vi "JKISM++ TCP Server SubModule(Beside Loop Support).vi"(7 "Name(\"\" to use uuid)":string="Event JKISM Tiny") -> ()   [LabVIEW 2014]
doc: "Demonstrates how to set up a basic TCP connection, send data to the specified port once a connection has been established, and terminate the connection once the data has been sent. This VI is designed to stop if the TCP connection is terminated. The data sent in this example is an array of random numbers."
uses:
  user.lib/_NEVSTOP/JKI State Machine++/_Support/JKISMQ/_Create Data Queue.vi
  user.lib/_NEVSTOP/JKI State Machine++/_Support/JKISMQ/_Obtain JKISMQ.vi
  user.lib/_NEVSTOP/JKI State Machine++/_Support/FGV-BroadcastRegistry/Cache-Broadcast Registry Search Result.vi
  user.lib/_NEVSTOP/JKI State Machine++/AdvanceAPI/JKISM++ Register Status Change.vi
  user.lib/_NEVSTOP/JKI State Machine++/AdvanceAPI/JKISM++ Unregister Status Change.vi
  user.lib/_NEVSTOP/JKI State Machine++/_Support/JKISMQ/_Create Resp Queue.vi
  user.lib/_NEVSTOP/JKI State Machine++/_Support/JKISMQ/_Unlock JKISMQ.vi
  user.lib/_NEVSTOP/JKI State Machine++/_Support/JKISMQ/_Lock State JKISMQ.vi
  user.lib/_NEVSTOP/JKI State Machine++/_Support/JKISMQ/_Release JKISMQ.vi
  user.lib/_NEVSTOP/JKI State Machine++/AdvanceAPI/JKISM++ Make String Arguments Safe.vi
  user.lib/_NEVSTOP/JKI State Machine++/_Support/JKISMQ/_Input Name to JKISM Mode.vi
  user.lib/_NEVSTOP/JKI State Machine++/Utility/uuid.vi
  user.lib/_NEVSTOP/JKI State Machine++/_Support/KeyWords.vi
  user.lib/_NEVSTOP/JKI State Machine++/_Support/JKISMQ/_JKISMQFGV.vi
  user.lib/_NEVSTOP/JKI State Machine++/_Support/GlobalEvent/FGV-GlobalEventRef.vi
  user.lib/_NEVSTOP/JKI State Machine++/_Support/JKISMQ/_Dequeue JKISMQ.vi
  user.lib/_NEVSTOP/JKI State Machine++/_Support/JKISMQ/_Enqueue JKISMQ.vi
  user.lib/_NEVSTOP/JKI State Machine++/_Support/GlobalEvent/FGV-StatusChangeEventRef.vi
  user.lib/_NEVSTOP/JKI State Machine++/_Support/FGV-BroadcastRegistry/global-Broadcast Cache Change Flag.vi
  user.lib/_NEVSTOP/JKI State Machine++/_Support/FGV-BroadcastRegistry/FGV-BroadcastRegistry.vi
  user.lib/_NEVSTOP/JKI State Machine++/JKI State Machine++.lvlib
panel:
  in  "Send String":string
  out "Connected":bool
  out "TCP Received":string
  out "TCP":refnum<k5>
  out "State History":string
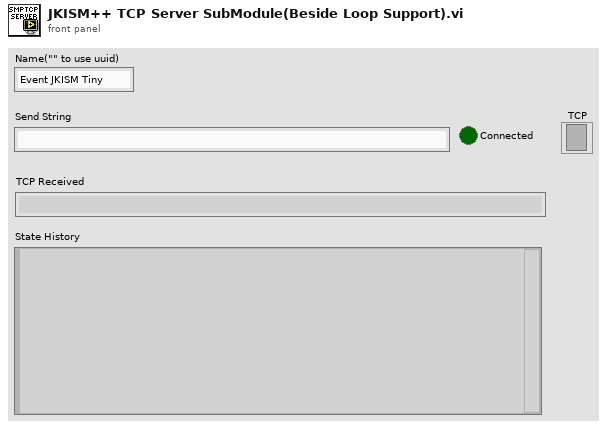
[diagram p1: front panel]
types:
  T1 = enum32{"Invalid", "Standard", "Closed", "Hidden", "Minimized", "Maximized"}
  T2 = enum32{"invalid app kind", "Development System", "Run Time System", "Student Edition", "Embedded LabVIEW", "Evaluation", "Custom"}
  T3 = cluster{"Core":cluster{"Current VI Reference":refnum<vi>, "Close Panel on Exit?":bool}, "Your Boolean data":bool, "Your string data":string}
  T4 = cluster{"Current VI Reference":refnum<vi>, "Close Panel on Exit?":bool}
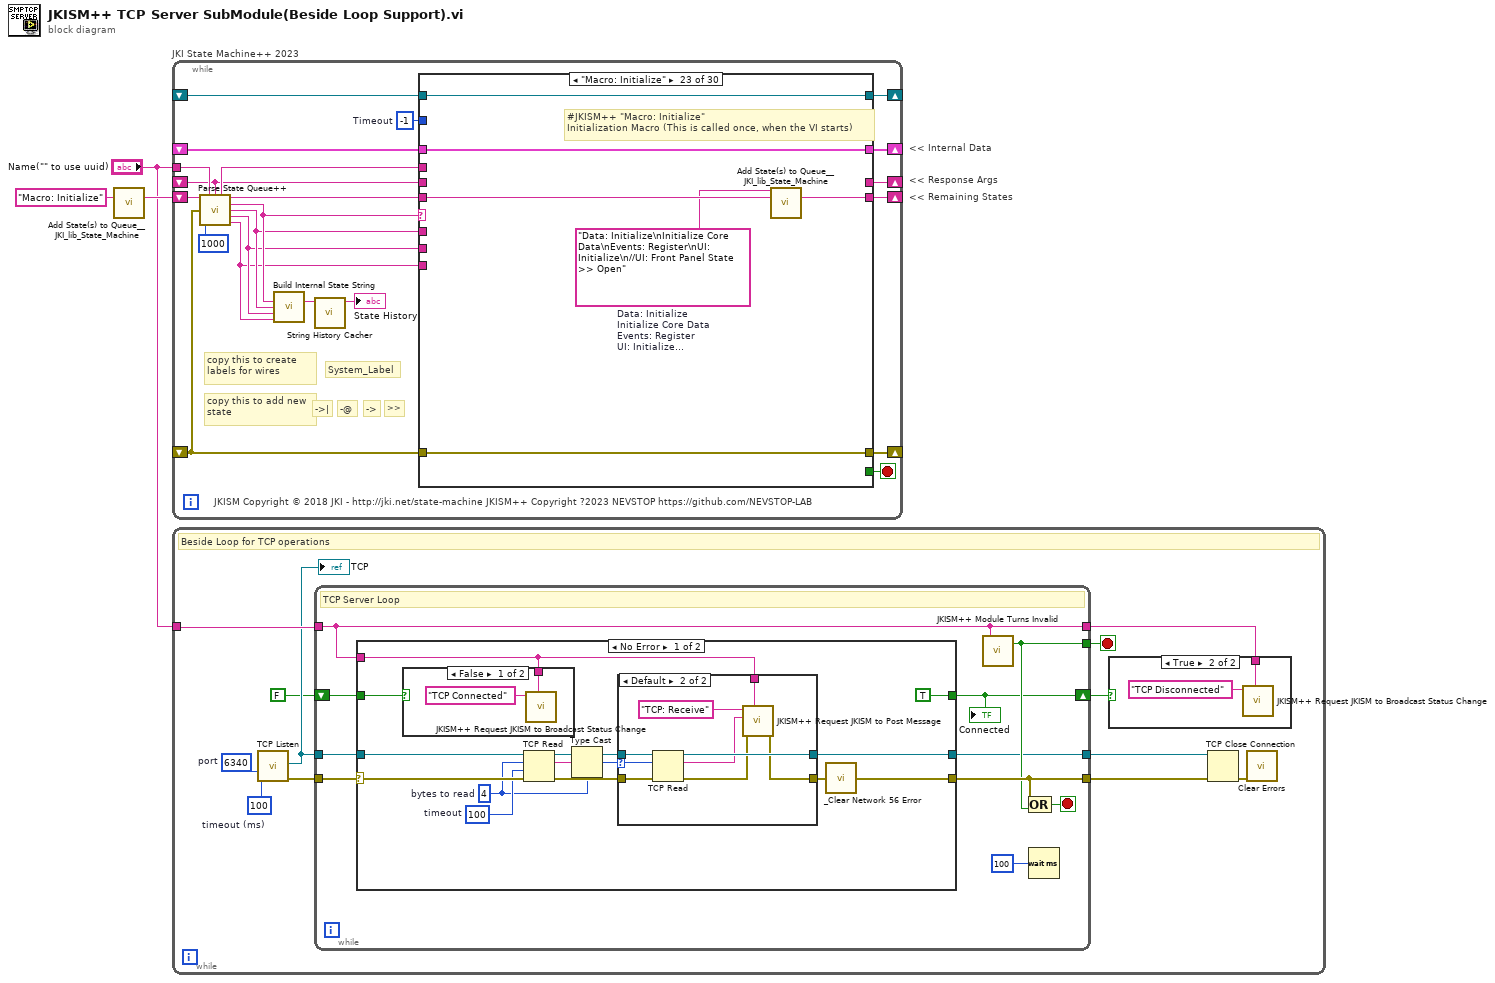
[diagram p0: block diagram]
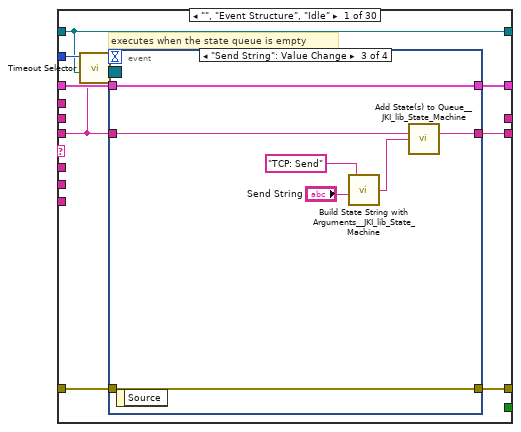
[diagram p2: hidden frame]
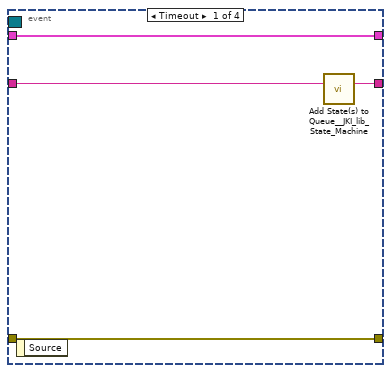
[diagram p3: hidden frame]
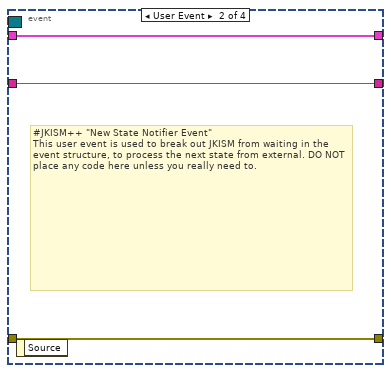
[diagram p4: hidden frame]
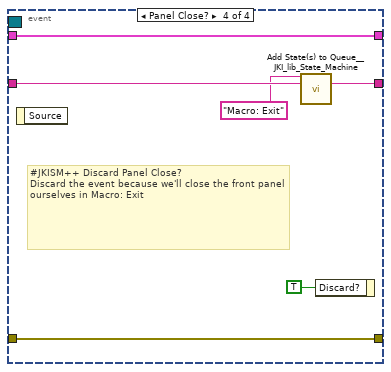
[diagram p5: hidden frame]
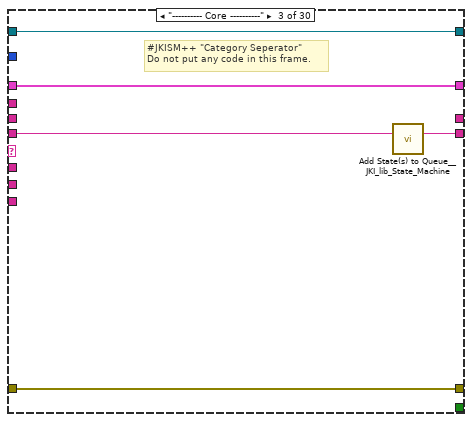
[diagram p7: hidden frame]
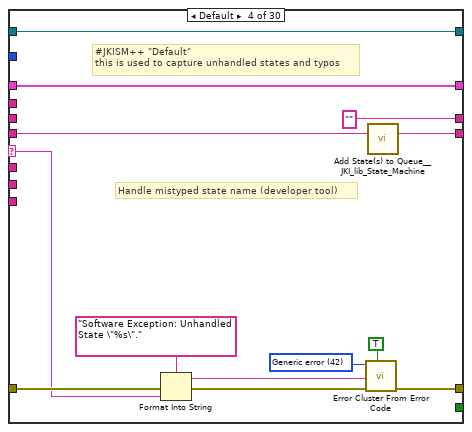
[diagram p8: hidden frame]
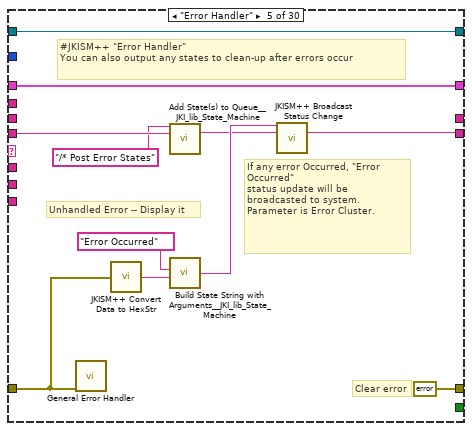
[diagram p9: hidden frame]
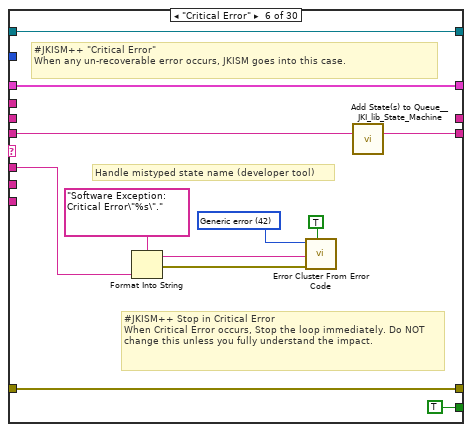
[diagram p10: hidden frame]
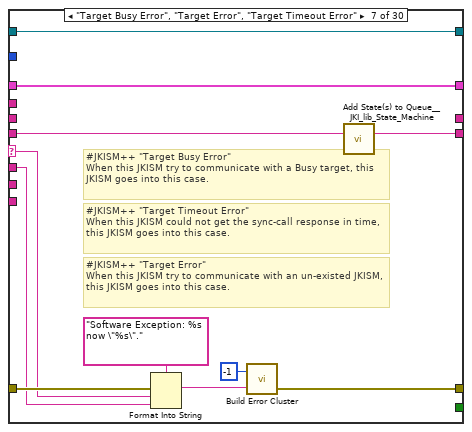
[diagram p11: hidden frame]
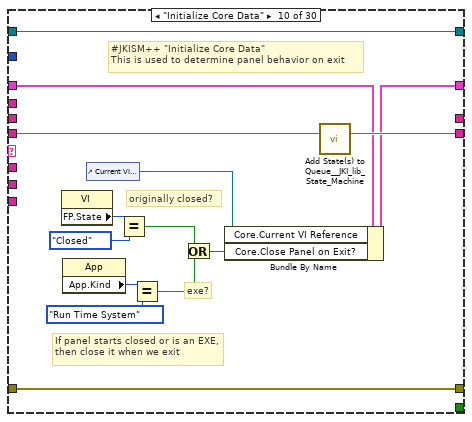
[diagram p14: hidden frame]
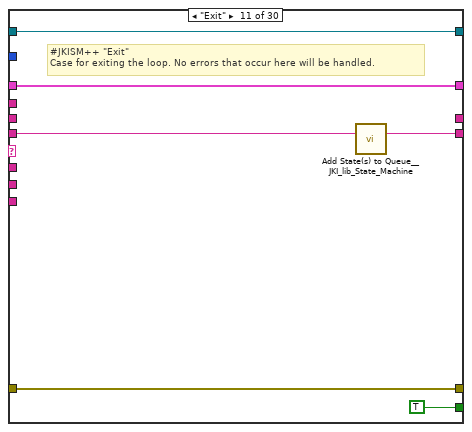
[diagram p15: hidden frame]
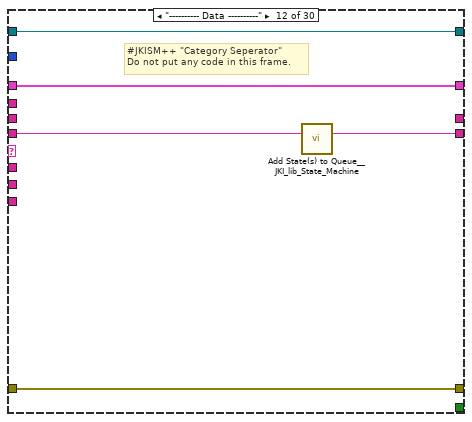
[diagram p16: hidden frame]
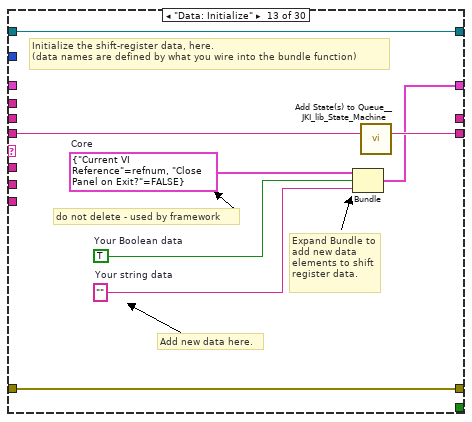
[diagram p17: hidden frame]
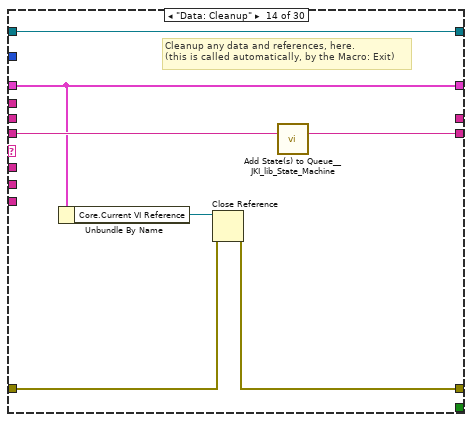
[diagram p18: hidden frame]
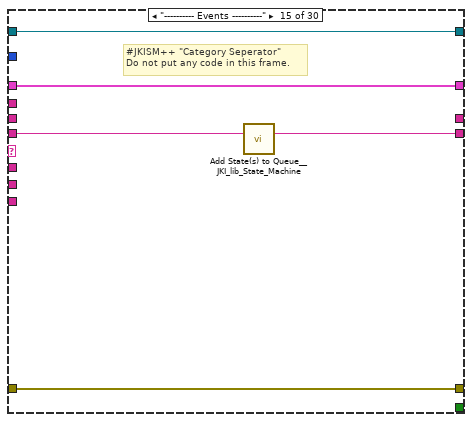
[diagram p19: hidden frame]
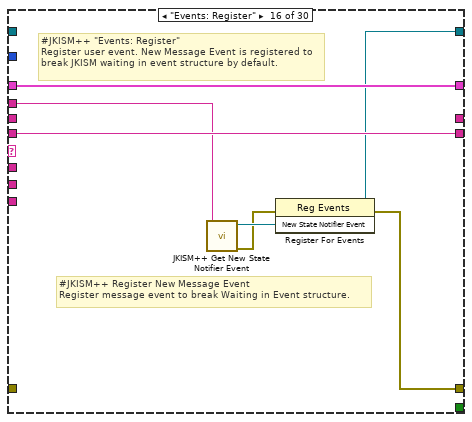
[diagram p20: hidden frame]
diagram:
  # "<< Internal Data"
  # "<< Response Args"
  # "<< Remaining States"
  n1 = call <vilib>:"Add State(s) to Queue__JKI_lib_State_Machine.vi"("State(s) in (\"\")"="Macro: Initialize") -> ("States Out"=w2:string)  [unwired: 14 in]
  n2 = while "JKI State Machine++ 2023" {
    shift-right: [w20] -> _
    shift-left: _ -> [w19]
    shift-right: [w23] -> _
    shift-left: _ -> [w17]
    shift-right: [w22] -> _
    shift-left: w2 -> [w24]
    tunnel: "Name(\"\" to use uuid)" -> [w12]
    shift-right: [w15] -> _
    shift-left: _ -> [w4]
    shift-right: [w14] -> _
    shift-left: _ -> [w13]
    stop <- w21 stop-if-true
    w18 = -1  # Timeout
    # "->|"
    # "JKISM Copyright © 2018 JKI - http://jki.net/state-machine JKISM++ Copyright ?2023 NEVSTOP https://github.com/NEVSTOP-LAB"
    # "copy this to add new state"
    # ">>"
    # "->"
    # "-@"
    # "copy this to create labels for wires"
    # "System_Label"
    n3 = call "Parse State Queue++.vi"("State Queue"=w24, "Name(\"\" to use uuid)"=w12, "Response Arguments"=w4, "Error In (no error)"=w17, "Response Timeout(5000ms)"=1000 ("Response Timeout(1000ms)")) -> ("Name Used"=w5:string, "Remaining States"=w25:string, "Current State"=w9:string, "Arguments"=w8:string, "Argument - State"=w7:string, "From Who"=w6:string)  [unwired: 5 in]
    n4 = call "Build Internal State String.vi"("State"=w9, "Arguments (\"\")"=w8, "Arg-State (\"\")"=w7, "Source (\"\")"=w6) -> ("State with Arguments"=w10:string)  [unwired: 11 in]
    n5 = call "String History Cacher.vi"("String"=w10) -> ("String Cache"=→"State History":string)  [unwired: 10 in]
    n6 = case shown="\"Macro: Initialize\"" w9 {
      selector: w9 -> [_ _ _ w66 _ _ w103 _ _ _ _ _ _ _ _ _ _ _ _ _ _ _ _ _ _ _ _ _ _ _]
      tunnel: w25 -> [w26 w57 w63 w70 w87 w97 w105 w113 w117 w132 w138 w143 w151 w158 w163 w170 w174 w180 w185 w192 w208 w278 w284 w295 w298 w309 w316 w322 w328 w334]
      tunnel: w8 -> [_ _ _ _ _ w90 w104 _ _ _ _ _ _ _ _ _ _ _ _ w187 w202 _ _ _ _ w300 w311 _ _ _]
      tunnel: w19 -> [w33 w56 w60 w68 w85 w98 w107 w112 w116 w125 w136 w140 _ w153 w160 w169 w173 w177 w183 w190 w204 w275 w281 w292 w297 w308 w315 w319 w325 w331]
      tunnel: [w32 w58 w61 w72 errorcluster {"status"=FALSE, "code"=0, "source"=""} ("error out") w99 w101 w114 w118 w129 w135 w141 w148 w154 w161 w164 w172 w178 w182 w188 w205 w276 w282 w293 w299 w301 w317 w320 w326 w332] -> w23
      tunnel: w17 -> [w31 w58 w61 w71 w77 w99 w109 w114 w118 w129 w135 w141 w148 w155 w161 _ w175 w178 w182 w189 w206 w276 w282 w293 w299 _ w317 w320 w326 w332]
      tunnel: [w34 w57 w62 w69 w78 w96 w108 w113 w117 w131 w137 w142 w150 w157 w162 w170 w174 w179 w184 w191 w207 w277 w283 w294 w298 w309 w313 w321 w327 w333] -> w22
      tunnel: [_ _ _ _ _ TRUE _ _ _ _ TRUE _ _ _ _ _ _ _ _ _ _ _ _ _ _ _ _ _ _ _] -> w21
      tunnel: [w30 w56 w60 w68 w85 w98 w107 w112 w116 w130 w136 w140 w149 w153 w160 w169 w173 w177 w183 w190 w204 w275 w281 w292 w297 w308 w315 w319 w325 w331] -> w20
      tunnel: w18 -> [w29 _ _ _ _ _ _ _ _ _ _ _ _ _ _ _ _ _ _ _ _ _ _ _ _ _ _ _ _ _]
      tunnel: w6 -> [_ _ _ _ _ _ _ _ _ _ _ _ _ _ _ _ _ _ _ _ _ _ _ _ _ _ _ _ _ _]
      tunnel: w7 -> [_ _ _ _ _ _ _ _ _ _ _ _ _ _ _ _ _ _ _ _ _ _ _ _ _ _ _ _ _ _]
      tunnel: [_ _ _ "" _ _ _ _ _ _ _ _ _ _ _ _ _ _ _ _ _ _ _ _ _ _ _ _ "DoA Finished" "DoB Finished"] -> w15
      tunnel: [w28 w55 w59 w64 w83 w88 w106 w111 w115 w119 w133 w139 w144 w152 w159 w168 w171 w176 w181 w186 w201 w274 w279 w285 w296 w307 w314 w318 w324 w330] -> w14
      tunnel: w13 -> [w28 w55 w59 w64 w83 w88 w106 w111 w115 w119 w133 w139 w144 w152 w159 _ w171 w176 w181 w186 w201 w274 w279 w285 w296 w307 w314 w318 w324 w330]
      tunnel: w5 -> [_ _ _ _ _ _ _ _ _ _ _ _ _ _ _ w167 _ _ _ _ _ _ _ _ _ _ _ _ _ _]
      tunnel: w4 -> [_ _ _ _ _ _ _ _ _ _ _ _ _ _ _ _ _ _ _ _ _ _ _ _ _ _ _ _ _ _]
      frame "", "Event Structure", "Idle" {
        # "executes when the state queue is empty"
        n7 = call "Timeout Selector.vi"("Remaining States"=w26, "Timeout Expected"=w29) -> ("Timeout"=w27:i32)  [unwired: 5 in]
        n8 = event shown="[2] \"Send String\": Value Change" {
          selector: w28 -> [_ _ _ _]
          dyn-events: _ -> [_ _ _ _]
          timeout: w27 -> [_ _ _ _]
          tunnel: w26 -> [w38 w40 w46 w54]
          tunnel: [w37 w40 w45 w53] -> w34
          tunnel: w33 -> [w35 w41 w47 w51]
          tunnel: [w36 w39 w48 w52] -> w32
          tunnel: w31 -> [w36 w39 w48 w52]
          tunnel: [w35 w41 w47 w51] -> w30
          event Timeout {
            n9 = event-data() -> ()  [unwired: 1 in, 1 out]
            n10 = call <vilib>:"Add State(s) to Queue__JKI_lib_State_Machine.vi"("State(s) in (\"\")"=w38) -> ("States Out"=w37:string)  [unwired: 14 in]
          }
          event User Event {
            # "#JKISM++ \"New State Notifier Event\"\nThis user event is used to break out JKISM from waiting in the event structure, to process the next state from external. DO NOT place any code here unless you really need to."
            n11 = event-data() -> ()  [unwired: 1 in, 1 out]
          }
          event "Send String": Value Change {
            n12 = event-data() -> ()  [unwired: 1 in, 1 out]
            n13 = call <vilib>:"Build State String with Arguments__JKI_lib_State_Machine.vi"("Arguments (\"\")"="Send String", "State"="TCP: Send") -> ("State with Arguments"=w43:string)  [unwired: 4 in]
            n14 = call <vilib>:"Add State(s) to Queue__JKI_lib_State_Machine.vi"("State(s) in (\"\")"=w46, "State(s) at Back (\"\")"=w43) -> ("States Out"=w45:string)  [unwired: 13 in]
          }
          event Panel Close? {
            # "#JKISM++ Discard Panel Close?\nDiscard the event because we'll close the front panel ourselves in Macro: Exit"
            n15 = event-data() -> ()  [unwired: 1 in, 1 out]
            n16 = call <vilib>:"Add State(s) to Queue__JKI_lib_State_Machine.vi"("State(s) in Front (\"\")"="Macro: Exit", "State(s) in (\"\")"=w54) -> ("States Out"=w53:string)  [unwired: 13 in]
            n17 = event-data("Discard?"=TRUE) -> ()  [unwired: 1 in, 1 out]
          }
        }
      }
      frame "JKISM++ Documentation" {
        # "#JKISM++ \"Documentation\"\nCase for holding JKISM++ Documenation"
      }
      frame "---------- Core ----------" {
        # "#JKISM++ \"Category Seperator\"\nDo not put any code in this frame."
        n18 = call <vilib>:"Add State(s) to Queue__JKI_lib_State_Machine.vi"("State(s) in (\"\")"=w63) -> ("States Out"=w62:string)  [unwired: 14 in]
      }
      frame Default {
        w75 = 42 items=["No error", "Argument error", "Memory is full", "Out of zone", "End of file", "File already open", "Generic file I/O error", "File not found", "File permission error", "Disk is full", "Duplicate path", "Too many files open", "System feature not enabled", "Resource file not found", "Cannot add resource", "Resource not found", "Image not found", "Image memory error", "Pen does not exist", "Config type invalid", "Config token not found", "Config parse error", "Config memory error", "Bad external code format", "Bad external code offset", "External code not present", "Null window", "Destroy window error", "Null menu", "Print aborted", "Bad print record", "Print driver error", "Windows error during printing", "Memory error during printing", "Print dialog error", "Generic print error", "Invalid device refnum", "Device not found", "Device parameter error", "Device unit error", "Cannot open device", "Device call aborted", "Generic error", "Cancelled by user", "Object ID too low", "Object ID too high", "Object not in heap", "Unknown heap", "Unknown object (invalid DefProc)", "Unknown object (DefProc not in table)", "Message out of range", "Invalid (null) method", "Unknown message", "Manager call not supported", "Bad address", "Network operation in progress", "Network operation timed out", "Connection is busy", "Network attribute not supported", "Network error", "Address in use", "System out of memory", "Connection aborted", "Connection refused", "Not connected", "Already connected", "Connection closed", "Initialization error (interapplication manager)", "Bad occurrence", "Wait on unbound occurrence handler", "Occurrence queue overflow", "Datalog type conflict", "Unused", "Unrecognized type (interapplication manager)", "Memory corrupt", "Failed to make temporary DLL", "Old CIN version", "Drag socket not found", "Failed to load drop-object", "Failed to register OLE object", "Failed to release OLE object", "Format specifier type mismatch", "Unknown format specifier", "Too few format specifiers", "Too many format specifiers", "Scan failed", "Newer CIN version", "Error converting to variant", "Runtime menu error", "Password tampered", "Variant attribute not found", "Incompatible variant data type", "Event data is not available", "Event Store is not present", "Occurrence is not found", "Event Queue is not created", "Event info is not available", "Refnum passed is NULL", "Error retrieving Class GUID", "Error retrieving CoClass GUID", "Error retrieving TypeLib GUID.", "Bad built application magic bytes.", "Specific driver is different from the specific driver associated with the Logical Name.", "There is no session opened to the class driver.", "Max Error", "MAX - Error with config objects", "MAX - Error loading configuration", "MAX - Group not supported"]
        # "#JKISM++ \"Default\"\nthis is used to capture unhandled states and typos"
        # "Handle mistyped state name (developer tool)"
        n19 = Format Into String(format string="Software Exception: Unhandled State \"%s\"." ("message"), error in=w71, w66) -> (resulting string=w74:string, error out=w73:errorcluster)  [unwired: 1 in]
        n20 = call <vilib>:"Error Cluster From Error Code.vi"("show call chain? (False)"=TRUE, "error in (no error)"=w73, "error message (\"\")"=w74, "error code (0)"=w75) -> ("error out"=w72:errorcluster)  [unwired: 5 in]
        n21 = call <vilib>:"Add State(s) to Queue__JKI_lib_State_Machine.vi"("State(s) in (\"\")"=w70) -> ("States Out"=w69:string)  [unwired: 14 in]
      }
      frame "Error Handler" {
        # "#JKISM++ \"Error Handler\"\nYou can also output any states to clean-up after errors occur"
        # "If any error Occurred, \"Error Occurred\" \nstatus update will be broadcasted to system.\nParameter is Error Cluster."
        # "Unhandled Error -- Display it"
        # "Clear error"
        n22 = call <vilib>:"General Error Handler.vi"("error in (no error)"=w77) -> ()  [unwired: 10 in, 5 out]
        n23 = call "JKISM++ Convert Data to HexStr.vi"("Variant"=w77) -> ("HEX String (0-9,A-F)"=w81:string)  [unwired: 8 in]
        n24 = call <vilib>:"Add State(s) to Queue__JKI_lib_State_Machine.vi"("State(s) in Front (\"\")"="/* Post Error States", "State(s) in (\"\")"=w87) -> ("States Out"=w79:string)  [unwired: 13 in]
        n25 = call <vilib>:"Build State String with Arguments__JKI_lib_State_Machine.vi"("Arguments (\"\")"=w81, "State"="Error Occurred" ("Status with Arguments")) -> ("State with Arguments"=w80:string)  [unwired: 4 in]
        n26 = call "JKISM++ Broadcast Status Change.vi"("Status with Arguments"=w80, "State Queue"=w79) -> ("Remaining States"=w78:string)  [unwired: 13 in]
      }
      frame "Critical Error" {
        w94 = 42 items=["No error", "Argument error", "Memory is full", "Out of zone", "End of file", "File already open", "Generic file I/O error", "File not found", "File permission error", "Disk is full", "Duplicate path", "Too many files open", "System feature not enabled", "Resource file not found", "Cannot add resource", "Resource not found", "Image not found", "Image memory error", "Pen does not exist", "Config type invalid", "Config token not found", "Config parse error", "Config memory error", "Bad external code format", "Bad external code offset", "External code not present", "Null window", "Destroy window error", "Null menu", "Print aborted", "Bad print record", "Print driver error", "Windows error during printing", "Memory error during printing", "Print dialog error", "Generic print error", "Invalid device refnum", "Device not found", "Device parameter error", "Device unit error", "Cannot open device", "Device call aborted", "Generic error", "Cancelled by user", "Object ID too low", "Object ID too high", "Object not in heap", "Unknown heap", "Unknown object (invalid DefProc)", "Unknown object (DefProc not in table)", "Message out of range", "Invalid (null) method", "Unknown message", "Manager call not supported", "Bad address", "Network operation in progress", "Network operation timed out", "Connection is busy", "Network attribute not supported", "Network error", "Address in use", "System out of memory", "Connection aborted", "Connection refused", "Not connected", "Already connected", "Connection closed", "Initialization error (interapplication manager)", "Bad occurrence", "Wait on unbound occurrence handler", "Occurrence queue overflow", "Datalog type conflict", "Unused", "Unrecognized type (interapplication manager)", "Memory corrupt", "Failed to make temporary DLL", "Old CIN version", "Drag socket not found", "Failed to load drop-object", "Failed to register OLE object", "Failed to release OLE object", "Format specifier type mismatch", "Unknown format specifier", "Too few format specifiers", "Too many format specifiers", "Scan failed", "Newer CIN version", "Error converting to variant", "Runtime menu error", "Password tampered", "Variant attribute not found", "Incompatible variant data type", "Event data is not available", "Event Store is not present", "Occurrence is not found", "Event Queue is not created", "Event info is not available", "Refnum passed is NULL", "Error retrieving Class GUID", "Error retrieving CoClass GUID", "Error retrieving TypeLib GUID.", "Bad built application magic bytes.", "Specific driver is different from the specific driver associated with the Logical Name.", "There is no session opened to the class driver.", "Max Error", "MAX - Error with config objects", "MAX - Error loading configuration", "MAX - Group not supported"]
        # "#JKISM++ Stop in Critical Error\nWhen Critical Error occurs, Stop the loop immediately. Do NOT change this unless you fully understand the impact."
        # "#JKISM++ \"Critical Error\"\nWhen any un-recoverable error occurs, JKISM goes into this case."
        # "Handle mistyped state name (developer tool)"
        n27 = Format Into String(format string="Software Exception: Critical Error\"%s\"." ("message"), w90) -> (resulting string=w93:string, error out=w92:errorcluster)  [unwired: 2 in]
        n28 = call <vilib>:"Error Cluster From Error Code.vi"("show call chain? (False)"=TRUE, "error in (no error)"=w92, "error message (\"\")"=w93, "error code (0)"=w94) -> ()  [unwired: 5 in, 1 out]
        n29 = call <vilib>:"Add State(s) to Queue__JKI_lib_State_Machine.vi"("State(s) in (\"\")"=w97) -> ("States Out"=w96:string)  [unwired: 14 in]
      }
      frame "Target Busy Error", "Target Error", "Target Timeout Error" {
        # "#JKISM++ \"Target Error\"\nWhen this JKISM try to communicate with an un-existed JKISM, this JKISM goes into this case."
        # "#JKISM++ \"Target Timeout Error\"\nWhen this JKISM could not get the sync-call response in time, this JKISM goes into this case."
        # "#JKISM++ \"Target Busy Error\"\nWhen this JKISM try to communicate with a Busy target, this JKISM goes into this case."
        n30 = Format Into String(format string="Software Exception: %s now \"%s\"." ("message"), error in=w109, w103, w104) -> (resulting string=w102:string)  [unwired: 1 in, 1 out]
        n31 = call "Build Error Cluster.vi"("String to Prepend to source (\"\")"=w102, "code"=-1) -> ("error out"=w101:errorcluster)
        n32 = call <vilib>:"Add State(s) to Queue__JKI_lib_State_Machine.vi"("State(s) in (\"\")"=w105) -> ("States Out"=w108:string)  [unwired: 14 in]
      }
      frame "Async Response", "Response" {
        # "#JKISM++ Response Comments\nAfter Message is executed, JKISM+ goes to this state for receive the response.\n    For Async Message(->), \"Async Response\" is used. This JKISM will goes to \"Async Message Posted\" immediately and receive the \"Async Response\" after the callee finishes the message.\n    For Sync Message(@),  This JKISM will wait until the message is done and immediately goes to \"Response\""
        # "#JKISM++ \"Async Response\"\nHandle Async-call Response (\"Async Response\" for ->)"
        # "#JKISM++ \"Response\"\nHandle Sync-call Response (\"Response\" for -@)"
      }
      frame "Async Message Posted" {
        # "#JKISM++ \"Async Message Posted\"\nAfter Async Message is posted (-> or ->| ), JKISM+ goes to this state for post-action.\nYou can use Argument - State to tell which Async Message is called."
      }
      frame "Initialize Core Data" {
        # "#JKISM++ \"Initialize Core Data\"\nThis is used to determine panel behavior on exit"
        # "originally closed?"
        # "exe?"
        # "If panel starts closed or is an EXE, then close it when we exit"
        n33 = property class="VI"() -> ("FP.State"=w122:T1)  [unwired: 2 in, 2 out]
        n34 = property class="App"() -> ("App.Kind"=w128:T2)  [unwired: 2 in, 2 out]
        n35 = control-ref of="Current VI Reference"() -> (w123:refnum<vi>)
        n36 = Equal?(x=w122, y=T1."Closed" ("Front Panel Window:State")) -> (x = y?=w120:bool)
        n37 = Equal?(x=w128, y=T2."Run Time System" ("Application:Kind")) -> (x = y?=w126:bool)
        n38 = Or(x=w120, y=w126) -> (x .or. y?=w124:bool)
        n39 = Bundle By Name(cluster=w125, "Core.Current VI Reference"=w123, "Core.Close Panel on Exit?"=w124) -> (w130:T3)
        n40 = call <vilib>:"Add State(s) to Queue__JKI_lib_State_Machine.vi"("State(s) in (\"\")"=w132) -> ("States Out"=w131:string)  [unwired: 14 in]
      }
      frame "Exit" {
        # "#JKISM++ \"Exit\"\nCase for exiting the loop. No errors that occur here will be handled."
        n41 = call <vilib>:"Add State(s) to Queue__JKI_lib_State_Machine.vi"("State(s) in (\"\")"=w138) -> ("States Out"=w137:string)  [unwired: 14 in]
      }
      frame "---------- Data ----------" {
        # "#JKISM++ \"Category Seperator\"\nDo not put any code in this frame."
        n42 = call <vilib>:"Add State(s) to Queue__JKI_lib_State_Machine.vi"("State(s) in (\"\")"=w143) -> ("States Out"=w142:string)  [unwired: 14 in]
      }
      frame "Data: Initialize" {
        w145 = T4 {"Current VI Reference"=refnum, "Close Panel on Exit?"=FALSE}  # Core
        w147 = TRUE  # Your Boolean data
        w146 = ""  # Your string data
        # "do not delete - used by framework"
        # "Expand Bundle to add new data elements to shift register data."
        # "Add new data here."
        # "Initialize the shift-register data, here.\n(data names are defined by what you wire into the bundle function)"
        n43 = Bundle("Core"=w145, "Your Boolean data"=w147, "Your string data"=w146) -> (w149:T3)  [unwired: 1 in]
        n44 = call <vilib>:"Add State(s) to Queue__JKI_lib_State_Machine.vi"("State(s) in (\"\")"=w151) -> ("States Out"=w150:string)  [unwired: 14 in]
      }
      frame "Data: Cleanup" {
        # "Cleanup any data and references, here.\n(this is called automatically, by the Macro: Exit)"
        n45 = Unbundle By Name(w153) -> ("Core.Current VI Reference"=w156:refnum<vi>)
        n46 = Close Reference(reference=w156, error in (no error)=w155) -> (error out=w154:errorcluster)
        n47 = call <vilib>:"Add State(s) to Queue__JKI_lib_State_Machine.vi"("State(s) in (\"\")"=w158) -> ("States Out"=w157:string)  [unwired: 14 in]
      }
      frame "---------- Events ----------" {
        # "#JKISM++ \"Category Seperator\"\nDo not put any code in this frame."
        n48 = call <vilib>:"Add State(s) to Queue__JKI_lib_State_Machine.vi"("State(s) in (\"\")"=w163) -> ("States Out"=w162:string)  [unwired: 14 in]
      }
      frame "Events: Register" {
        # "#JKISM++ \"Events: Register\"\nRegister user event. New Message Event is registered to break JKISM waiting in event structure by default."
        # "#JKISM++ Register New Message Event\nRegister message event to break Waiting in Event structure."
        n49 = call "JKISM++ Get New State Notifier Event.vi"("Name(\"\" to use uuid) in"=w167) -> ("Error out"=w165:errorcluster, "New State Notifier Event"=w166:refnum<user-event>)  [unwired: 9 in]
        n50 = register-events(error in=w165, w166) -> (reference out=w168:refnum<event-registration>, error out=w164:errorcluster)  [unwired: 1 in]
      }
      frame "Events: Unregister" {
        # "#JKISM++ \"Events: Unregister\"\nUnregister user event."
        n51 = Unregister For Events(event registration refnum=w171, error in=w175) -> (error out=w172:errorcluster)
      }
      frame "---------- UI ----------" {
        # "#JKISM++ \"Category Seperator\"\nDo not put any code in this frame."
        n52 = call <vilib>:"Add State(s) to Queue__JKI_lib_State_Machine.vi"("State(s) in (\"\")"=w180) -> ("States Out"=w179:string)  [unwired: 14 in]
      }
      frame "UI: Initialize" {
        # "#JKISM++ \"UI: Initialize\"\nInitialize the User Interface, here.\n(this is called automatically, by the Macro: Init)"
        n53 = call <vilib>:"Add State(s) to Queue__JKI_lib_State_Machine.vi"("State(s) in (\"\")"=w185) -> ("States Out"=w184:string)  [unwired: 14 in]
      }
      frame "UI: Cursor Set" {
        # "#JKISM++ \"UI: Cursor Set\"\nSet and Unset Cursor Busy.\n(Usage: \"UI: Cursor Set >> Busy|Idle\")"
        # "Argument"
        n54 = disable-structure shown="TARGET_TYPE!=Windows" {
          disable-tunnel: w189 -> [w195 w200]
          disable-tunnel: [w194 w200] -> w188
          disable-tunnel: w187 -> [w193 _]
          frame condition #0 (active) {
            n55 = case shown="\"Idle\", Default" w193 {
              tunnel: w195 -> [w197 w199]
              tunnel: [w196 w198] -> w194
              frame "Idle", Default {
                n56 = call <vilib>:"Unset Busy.vi"("error in (no error)"=w197) -> ("error out"=w196:errorcluster)  [unwired: 10 in]
              }
              frame "Busy" {
                n57 = call <vilib>:"Set Busy.vi"("error in (no error)"=w199) -> ("error out"=w198:errorcluster)  [unwired: 9 in, 1 out]
              }
            }
          }
          frame condition #1 {
          }
        }
        n58 = call <vilib>:"Add State(s) to Queue__JKI_lib_State_Machine.vi"("State(s) in (\"\")"=w192) -> ("States Out"=w191:string)  [unwired: 14 in]
      }
      frame "UI: Front Panel State" {
        # "#JKISM++ \"UI: Front Panel State\"\nSet Front Panel Open or Closed\n(Usage: \"UI: Front Panel State >> Open|Close\")"
        # "Argument"
        n59 = Unbundle By Name(w204) -> ("Core.Current VI Reference"=w203:refnum<vi>)
        n60 = call <vilib>:"Add State(s) to Queue__JKI_lib_State_Machine.vi"("State(s) in (\"\")"=w208) -> ("States Out"=w207:string)  [unwired: 14 in]
        n61 = case shown="\"Close\", \"Closed\"" w202 {
          tunnel: w206 -> [w214 w229 w240 w253 w266]
          tunnel: [w216 w230 w242 w255 w268] -> w205
          tunnel: w203 -> [w215 w227 w241 w254 w267]
          frame "Open", "Standard", Default {
            w209 = T1."Standard" ("State")
            n62 = property class="VI"(reference=w215, error in=w214) -> (reference out=w212:refnum<vi>, error out=w213:errorcluster, "FP.State"=w211:T1)
            n63 = Not Equal?(x=w211, y=w209) -> (x != y?=w210:bool)
            n64 = case shown="True" w210 {
              tunnel: [w220 w222] -> w216
              tunnel: w213 -> [w219 w222]
              tunnel: w212 -> [w218 _]
              tunnel: w209 -> [w217 _]
              frame True {
                n65 = invoke class="VI" method="FP.Open"(reference=w218, error in=w219, "Activate"=TRUE, "State"=w217) -> (error out=w220:errorcluster)  [unwired: 1 in, 4 out]
              }
              frame False {
              }
            }
          }
          frame "Close", "Closed" {
            n66 = property class="VI"(reference=w227, error in=w229) -> (reference out=w226:refnum<vi>, error out=w228:errorcluster, "FP.State"=w224:T1)
            n67 = Not Equal?(x=w224, y=T1."Closed" ("Front Panel Window:State")) -> (x != y?=w223:bool)
            n68 = case shown="False" w223 {
              tunnel: [w231 w234] -> w230
              tunnel: w228 -> [w231 w233]
              tunnel: w226 -> [_ w232]
              frame False {
              }
              frame True {
                n69 = invoke class="VI" method="FP.Close"(reference=w232, error in=w233) -> (error out=w234:errorcluster)  [unwired: 1 in, 2 out]
              }
            }
          }
          frame "Hidden", "Hide" {
            w235 = T1."Hidden" ("State")
            n70 = property class="VI"(reference=w241, error in=w240) -> (reference out=w238:refnum<vi>, error out=w239:errorcluster, "FP.State"=w237:T1)
            n71 = Not Equal?(x=w237, y=w235) -> (x != y?=w236:bool)
            n72 = case shown="True" w236 {
              tunnel: [w246 w247] -> w242
              tunnel: w239 -> [w245 w247]
              tunnel: w238 -> [w244 _]
              tunnel: w235 -> [w243 _]
              frame True {
                n73 = invoke class="VI" method="FP.Open"(reference=w244, error in=w245, "State"=w243) -> (error out=w246:errorcluster)  [unwired: 2 in, 4 out]
              }
              frame False {
              }
            }
          }
          frame "Minimize", "Minimized" {
            w248 = T1."Minimized" ("State")
            n74 = property class="VI"(reference=w254, error in=w253) -> (reference out=w251:refnum<vi>, error out=w252:errorcluster, "FP.State"=w250:T1)
            n75 = Not Equal?(x=w250, y=w248) -> (x != y?=w249:bool)
            n76 = case shown="True" w249 {
              tunnel: [w259 w260] -> w255
              tunnel: w252 -> [w258 w260]
              tunnel: w251 -> [w257 _]
              tunnel: w248 -> [w256 _]
              frame True {
                n77 = invoke class="VI" method="FP.Open"(reference=w257, error in=w258, "State"=w256) -> (error out=w259:errorcluster)  [unwired: 2 in, 4 out]
              }
              frame False {
              }
            }
          }
          frame "Maximize", "Maximized" {
            w261 = T1."Maximized" ("State")
            n78 = property class="VI"(reference=w267, error in=w266) -> (reference out=w264:refnum<vi>, error out=w265:errorcluster, "FP.State"=w263:T1)
            n79 = Not Equal?(x=w263, y=w261) -> (x != y?=w262:bool)
            n80 = case shown="True" w262 {
              tunnel: [w272 w273] -> w268
              tunnel: w265 -> [w271 w273]
              tunnel: w264 -> [w270 _]
              tunnel: w261 -> [w269 _]
              frame True {
                n81 = invoke class="VI" method="FP.Open"(reference=w270, error in=w271, "State"=w269) -> (error out=w272:errorcluster)  [unwired: 2 in, 4 out]
              }
              frame False {
              }
            }
          }
        }
      }
      frame "---------- Macro ----------" {
        # "#JKISM++ \"Category Seperator\"\nDo not put any code in this frame."
        n82 = call <vilib>:"Add State(s) to Queue__JKI_lib_State_Machine.vi"("State(s) in (\"\")"=w278) -> ("States Out"=w277:string)  [unwired: 14 in]
      }
      frame "Macro: Initialize" {
        w280 = "Data: Initialize\nInitialize Core Data\nEvents: Register\nUI: Initialize\n//UI: Front Panel State >> Open"  # Data: Initialize Initialize Core Data Events: Register UI: Initialize //UI: Front Panel State >> Open
        # "#JKISM++ \"Macro: Initialize\"\nInitialization Macro (This is called once, when the VI starts)"
        n83 = call <vilib>:"Add State(s) to Queue__JKI_lib_State_Machine.vi"("State(s) in Front (\"\")"=w280, "State(s) in (\"\")"=w284) -> ("States Out"=w283:string)  [unwired: 13 in]
      }
      frame "Macro: Exit" {
        # "#JKISM++ \"Macro: Exit\"\nExit Macro (This is called once, when the VI exits)"
        n84 = Unbundle By Name(w292) -> ("Core.Close Panel on Exit?"=w291:bool)
        n85 = Select(t="UI: Front Panel State >> Close", s=w291, f="") -> (s? t:f=w288:string)
        n86 = call <vilib>:"Add State(s) to Queue__JKI_lib_State_Machine.vi"("State(s) in (\"\")"=w288, "State(s) at Back (\"\")"="Data: Cleanup\nEvents: Unregister\nExit") -> ("States Out"=w286:string)  [unwired: 13 in]
        n87 = call <vilib>:"Add State(s) to Queue__JKI_lib_State_Machine.vi"("State(s) in Front (\"\")"=w286, "State(s) in (\"\")"=w295) -> ("States Out"=w294:string)  [unwired: 13 in]
      }
      frame "---------- API ----------" {
        # "#JKISM++ \"Category Seperator\"\nDo not put any code in this frame."
      }
      frame "TCP: Send" {
        n88 = local read "TCP"() -> (w302:refnum<k5>)
        n89 = String Length(string=w300) -> (length=w304:i32)
        n90 = Type Cast(x=w304) -> (*(type *) &x=w303:string)  [unwired: 1 out]
        n91 = TCP Write(connection ID=w302, data in=w303) -> (connection ID out=w306:refnum<k5>, error out=w305:errorcluster)  [unwired: 1 in, 2 out]
        n92 = TCP Write(connection ID=w306, data in=w300, error in (no error)=w305) -> (error out=w301:errorcluster)  [unwired: 3 out]
      }
      frame "TCP: Receive" {
        n93 = call <vilib>:"Build State String with Arguments__JKI_lib_State_Machine.vi"("Arguments (\"\")"=w311, "State"="TCP Received") -> ("State with Arguments"=w310:string)  [unwired: 4 in]
        n94 = call "JKISM++ Broadcast Status Change.vi"("Status with Arguments"=w310, "State Queue"=w316) -> ("Remaining States"=w313:string)  [unwired: 13 in]
        "TCP Received" <- w311
      }
      frame "---------- DoSth ----------" {
        # "#JKISM++ \"Category Seperator\"\nDo not put any code in this frame."
        n95 = call <vilib>:"Add State(s) to Queue__JKI_lib_State_Machine.vi"("State(s) in (\"\")"=w322) -> ("States Out"=w321:string)  [unwired: 14 in]
      }
      frame "DoSth: DoA" {
        # "#JKISM++ \"Internal State\"\nThis category is used for holding internal states"
        n96 = call <vilib>:"Add State(s) to Queue__JKI_lib_State_Machine.vi"("State(s) in (\"\")"=w328) -> ("States Out"=w327:string)  [unwired: 14 in]
      }
      frame "DoSth: DoB" {
        # "#JKISM++ \"Internal State\"\nThis category is used for holding internal states"
        n97 = call <vilib>:"Add State(s) to Queue__JKI_lib_State_Machine.vi"("State(s) in (\"\")"=w334) -> ("States Out"=w333:string)  [unwired: 14 in]
      }
    }
  }
  n98 = while {
    tunnel: "Name(\"\" to use uuid)" -> [w341]
    stop <- w342 stop-if-true
    w343 = u16 6340  # port
    w344 = 100  # timeout (ms)
    # "Beside Loop for TCP operations"
    n99 = call <vilib>:"TCP Listen.vi"("timeout ms (wait forever: -1)"=w344, "port"=w343) -> ("error out"=w345:errorcluster, "connection ID"=w340:refnum<k5>)  [unwired: 5 in, 3 out]
    "TCP" <- w340
    n100 = while {
      tunnel: [w356] -> w337
      tunnel: [w352] -> w346
      tunnel: w340 -> [w354]
      tunnel: w345 -> [w353]
      tunnel: [w355] -> w342
      tunnel: w341 -> [w350]
      tunnel: [w350] -> w338
      shift-right: [w349] -> w335
      shift-left: FALSE -> [w351]
      stop <- w357 stop-if-true
      # "TCP Server Loop"
      n101 = case shown="No Error" w353 {
        selector: w353 -> [w370 w388]
        tunnel: [w372 w388] -> w356
        tunnel: w354 -> [w371 w387]
        tunnel: [w367 w387] -> w352
        tunnel: w351 -> [w361 _]
        tunnel: w350 -> [w362 _]
        tunnel: [TRUE FALSE] -> w349
        frame No Error {
          w364 = 100  # timeout
          w359 = 4  # bytes to read
          n102 = case shown="False" w361 {
            tunnel: w362 -> [w385 _]
            frame False {
              n103 = call "JKISM++ Request JKISM to Broadcast Status Change.vi"("Module Name"=w385, "Status"="TCP Connected") -> ()  [unwired: 9 in, 1 out]
            }
            frame True {
            }
          }
          n104 = TCP Read(connection ID=w371, bytes to read=w359, error in (no error)=w370, 9:w364) -> (connection ID out=w368:refnum<k5>, data out=w366:string, error out=w369:errorcluster)  [unwired: 1 out]
          n105 = Type Cast(type=w359, x=w366) -> (*(type *) &x=w365:i32)
          n106 = case shown="Default" w365 {
            selector: w365 -> [_ w380]
            tunnel: w369 -> [w373 w383]
            tunnel: w368 -> [w374 w382]
            tunnel: [w374 w381] -> w367
            tunnel: [w373 w376] -> w363
            tunnel: w362 -> [_ w375]
            frame 0 {
            }
            frame Default {
              n107 = TCP Read(connection ID=w382, bytes to read=w380, error in (no error)=w383) -> (connection ID out=w381:refnum<k5>, data out=w379:string, error out=w377:errorcluster)  [unwired: 2 out]
              n108 = call "JKISM++ Request JKISM to Post Message.vi"("Module Name"=w375, "Error In (no error)"=w377, "Arguments (\"\")"=w379, "State"="TCP: Receive") -> ("error out"=w376:errorcluster)  [unwired: 7 in]
            }
          }
          n109 = call "_Clear Network 56 Error.vi"("error in (no error)"=w363) -> ("error out"=w372:errorcluster)  [unwired: 4 in]
        }
        frame Error {
        }
      }
      "Connected" <- w349
      n110 = call "JKISM++ Module Turns Invalid.vi"("JKISM Name"=w350) -> ("Turn Invalid(Exit)?"=w355:bool)  [unwired: 2 in]
      n111 = Compound Arithmetic op=OR(w356, w355) -> (w357:bool)
      n112 = Wait (ms)(milliseconds to wait=u32 100) -> ()  [unwired: 1 out]
    }
    n113 = case shown="True" w335 {
      tunnel: w338 -> [_ w348]
      frame False {
      }
      frame True {
        n114 = call "JKISM++ Request JKISM to Broadcast Status Change.vi"("Module Name"=w348, "Status"="TCP Disconnected") -> ()  [unwired: 9 in, 1 out]
      }
    }
    n115 = TCP Close Connection(connection ID=w346, error in (no error)=w337) -> (error out=w339:errorcluster)  [unwired: 2 out]
    n116 = call <vilib>:"Clear Errors.vi"("error in (no error)"=w339) -> ()  [unwired: 6 in, 1 out]
  }
